vi "Do.vi"(8 "error in (no error)":errorcluster, 10 "Actor in":refnum<class "Actor.lvclass">, 11 "WernerReadback Msg":refnum<class "Update_Readback Msg.lvclass">) -> (0 "error out":errorcluster, 2 "Actor out":refnum<class "Actor.lvclass">)   [LabVIEW 2015, in "CS++IEFWerner.lvlib" / "Update_Readback Msg.lvclass"]
doc: "This VI delivers the message to the actor by calling the appropriate method(s) on the actor."
uses:
  Update_Readback Msg.lvclass
  <vilib>/ActorFramework/Actor/Actor.lvclass
  CS++IEFWerner/CS++IEFWerner.lvclass
  CSPP_Core/Actors/CS++PVMonitor Messages/CS++PVUpdate Msg/CS++PVUpdate Msg.lvclass/CS++PVUpdate Msg.ctl
  Update_Readback Msg.lvclass/Update_Readback Msg.ctl
  CSPP_Core/Classes/CS++ProcessVariables/ProcessVariable/PV.lvclass/PV.ctl
  CSPP_Core/Classes/CS++ProcessVariables/ProcessVariable/PV.lvclass
  CSPP_Core/Actors/CS++PVMonitor Messages/CS++PVUpdate Msg/CS++PVUpdate Msg.lvclass
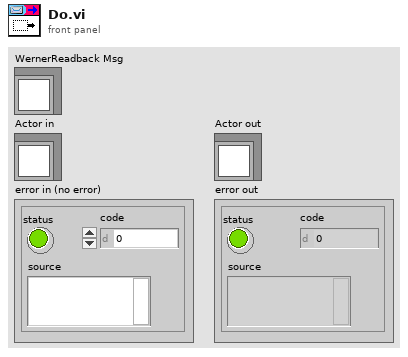
[diagram p1: front panel]
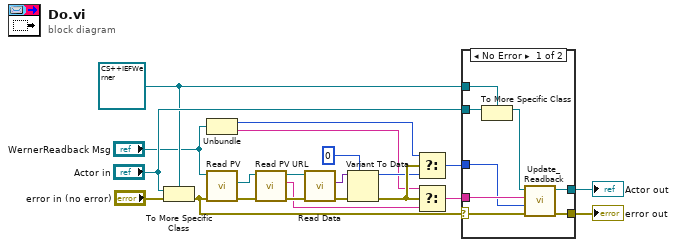
[diagram p0: block diagram]
diagram:
  w17 = refnum<class "CS++IEFWerner.lvclass"> refnum ("Actor in")
  n1 = To More Specific Class(target class=w17, reference="Actor in", error in="error in (no error)") -> (error out=w9:errorcluster)  [unwired: 1 out]
  n2 = Unbundle("WernerReadback Msg") -> (w2:u32, w1:string)
  n3 = call "Read PV.vi"("error in (no error)"=w9, "CS++PVUpdate Msg in"="WernerReadback Msg") -> ("error out"=w14:errorcluster, "PV"=w12:refnum<class "PV.lvclass">)  [unwired: 7 in, 1 out]
  n4 = call "Read PV URL.vi"("error in (no error)"=w14, "PV in"=w12) -> ("error out"=w13:errorcluster, "PV URL"=w7:string, "PV out"=w11:refnum<class "PV.lvclass">)  [unwired: 7 in]
  n5 = call "Read Data.vi"("error in (no error)"=w13, "PV in"=w11) -> ("error out"=w15:errorcluster, "Data"=w16:variant)  [unwired: 7 in, 1 out]
  n6 = Variant To Data(error in=w15, type=u32 0 ("Value"), Variant=w16) -> (data=w5:u32, error out=w8:errorcluster)
  n7 = Select(t=w2, s=w8, f=w5) -> (s? t:f=w4:u32)
  n8 = Select(t=w1, s=w8, f=w7) -> (s? t:f=w6:string)
  n9 = case shown="No Error" w9 {
    selector: w9 -> [w27 w31]
    tunnel: [w29 w31] -> w20
    tunnel: [w28 w30] -> w19
    tunnel: "Actor in" -> [w26 w30]
    tunnel: w17 -> [w25 _]
    tunnel: w6 -> [w23 _]
    tunnel: w4 -> [w22 _]
    frame No Error {
      n10 = To More Specific Class(target class=w25, reference=w26) -> (specific class reference=w24:refnum<class "CS++IEFWerner.lvclass">)  [unwired: 1 in, 1 out]
      n11 = call "Update_Readback.vi"("error in (no error)"=w27, "Value"=w22, "PV URL"=w23, "CS++IEFWerner in"=w24) -> ("error out"=w29:errorcluster, "CS++IEFWerner out"=w28:refnum<class "CS++IEFWerner.lvclass">)  [unwired: 6 in]
    }
    frame Error {
    }
  }
  "error out" <- w20
  "Actor out" <- w19
